vi "Send_Waypoints.vi"() -> ()   [LabVIEW 2009]
uses:
  <vilib>/Instr/_visa.llb/VISA Configure Serial Port (Instr).vi
panel:
  out "Waypoints Received":bool
  out "WRITE BUFFER":string
  out "READ BUFFER":string
  out "error out":errorcluster
  in  "baud rate":u32=115200
  in  "VISA resource name":refnum<visa-resource-name>
  in  "stop":bool
  in  "Request Type":enum16{"Append to End", "Replace List"}(ring)
  in  "Waypoint List":T1(array[cluster])=[{"Latitude"=29.316231, "Longitude"=-81.345678, "Altitude"=100}] {"Longitude" format="%#_15g"; "Latitude" format="%#_15g"}
  in  "Send Waypoints":bool
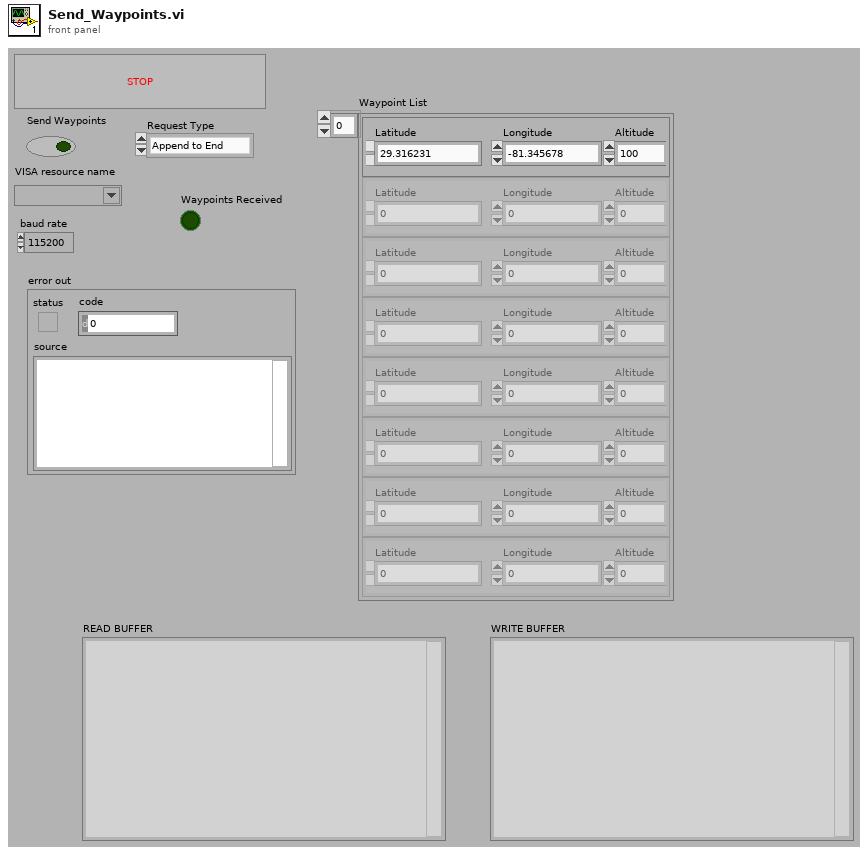
[diagram p1: front panel]
types:
  T1 = cluster{"Latitude":dbl, "Longitude":dbl, "Altitude":u16}[]
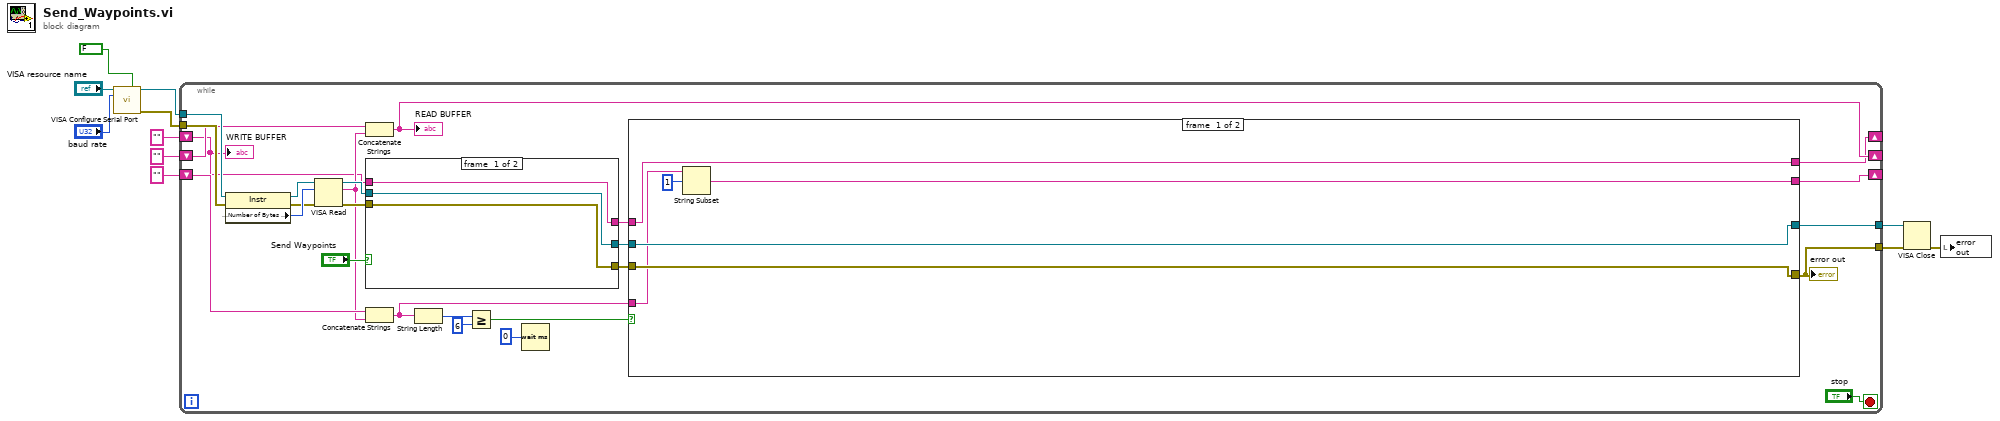
[diagram p0: block diagram]
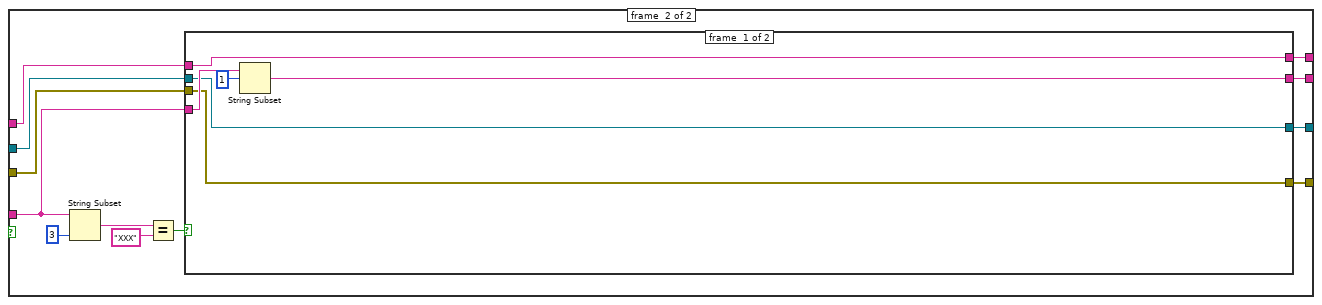
[diagram p2: hidden frame]
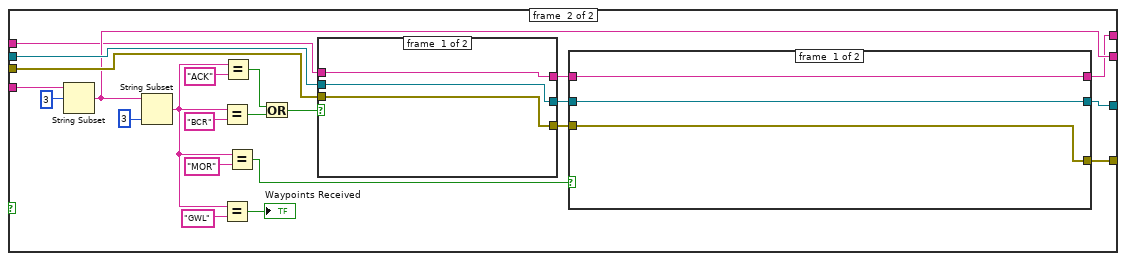
[diagram p3: hidden frame]
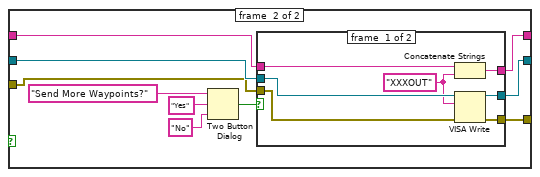
[diagram p4: hidden frame]
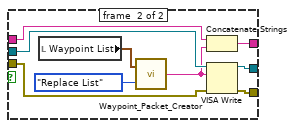
[diagram p5: hidden frame]
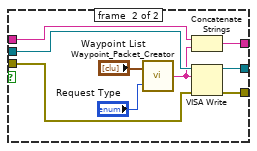
[diagram p6: hidden frame]
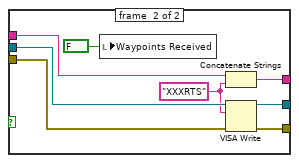
[diagram p7: hidden frame]
diagram:
  n1 = call-poly "VISA Configure Serial Port"("VISA resource name"="VISA resource name", "Enable Termination\nChar (T)"=FALSE ("Enable Termination\nChar (T)"), "baud rate (9600)"="baud rate") -> ("VISA resource name out"=w11:refnum<visa-resource-name>, "error out"=w7:errorcluster)  [unwired: 11 in]
  n2 = while {
    tunnel: w11 -> [w35]
    tunnel: w7 -> [w34]
    shift-right: [w24] -> _
    shift-left: "" -> [w30]
    tunnel: [w21] -> w5
    tunnel: [w20] -> w4
    shift-right: [w15] -> _
    shift-left: "" -> [w17]
    shift-right: [w12] -> _
    shift-left: "" -> [w14]
    stop <- "stop" stop-if-true
    n3 = property class="Instr"(reference=w35, error in=w34) -> (reference out=w33:refnum<visa-resource-name>, error out=w31:errorcluster, "Serial Settings:Number of Bytes at Serial Port"=w32:u32)
    n4 = VISA Read(VISA resource name=w33, byte count=w32, error in (no error)=w31) -> (VISA resource name out=w29:refnum<visa-resource-name>, read buffer=w16:string, error out=w28:errorcluster)  [unwired: 1 out]
    n5 = Concatenate Strings(w17, w16) -> (w15:string)
    "READ BUFFER" <- w15
    n6 = case shown="True" "Send Waypoints" {
      tunnel: w29 -> [w128 w136]
      tunnel: w28 -> [w127 w135]
      tunnel: [w127 w134] -> w22
      tunnel: [w128 w133] -> w23
      tunnel: w14 -> [w126 w131]
      tunnel: [w126 w130] -> w13
      frame #0 {
      }
      frame #1 {
        w132 = "XXXRTS" ("write buffer")
        n7 = local write "Waypoints Received"(FALSE ("Waypoints Received")) -> ()
        n8 = Concatenate Strings(w131, w132) -> (w130:string)
        n9 = VISA Write(VISA resource name=w136, write buffer=w132, error in (no error)=w135) -> (VISA resource name out=w133:refnum<visa-resource-name>, error out=w134:errorcluster)  [unwired: 1 out]
      }
    }
    n10 = Concatenate Strings(w30, w16) -> (w18:string)
    n11 = String Length(string=w18) -> (length=w27:i32)
    n12 = Greater Or Equal?(x=w27, y=6) -> (x >= y?=w25:bool)
    n13 = Wait (ms)(milliseconds to wait=u32 0) -> ()  [unwired: 1 out]
    n14 = case shown="True" w25 {
      tunnel: w18 -> [w41 w51]
      tunnel: [w40 w50] -> w24
      tunnel: w23 -> [w43 w49]
      tunnel: w22 -> [w42 w48]
      tunnel: [w43 w47] -> w21
      tunnel: [w42 w46] -> w20
      tunnel: w13 -> [w38 w45]
      tunnel: [w38 w44] -> w12
      frame #0 {
        n15 = String Subset(string=w41, offset (0)=1 ("length (rest)")) -> (substring=w40:string)  [unwired: 1 in]
      }
      frame #1 {
        n16 = String Subset(string=w51, length (rest)=3 ("length (rest)")) -> (substring=w54:string)  [unwired: 1 in]
        n17 = Equal?(x=w54, y="XXX") -> (x = y?=w52:bool)
        n18 = case shown="True" w52 {
          tunnel: w51 -> [w61 w80]
          tunnel: [w59 w69] -> w50
          tunnel: w49 -> [w58 w78]
          tunnel: w48 -> [w57 w77]
          tunnel: [w58 w71] -> w47
          tunnel: [w57 w70] -> w46
          tunnel: w45 -> [w56 w68]
          tunnel: [w56 w66] -> w44
          frame #0 {
            n19 = String Subset(string=w61, offset (0)=1) -> (substring=w59:string)  [unwired: 1 in]
          }
          frame #1 {
            n20 = String Subset(string=w80, offset (0)=3) -> (substring=w69:string)  [unwired: 1 in]
            n21 = String Subset(string=w69, length (rest)=3 ("length (rest)")) -> (substring=w64:string)  [unwired: 1 in]
            n22 = Equal?(x=w64, y="BCR") -> (x = y?=w63:bool)
            n23 = Equal?(x=w64, y="GWL") -> (x = y?=→"Waypoints Received":bool)
            n24 = Equal?(x=w64, y="ACK") -> (x = y?=w76:bool)
            n25 = Equal?(x=w64, y="MOR") -> (x = y?=w74:bool)
            n26 = Or(x=w76, y=w63) -> (x .or. y?=w75:bool)
            n27 = case shown="True" w75 {
              tunnel: w78 -> [w116 w123]
              tunnel: w77 -> [w115 w122]
              tunnel: [w116 w121] -> w73
              tunnel: [w115 w120] -> w72
              tunnel: w68 -> [w114 w119]
              tunnel: [w114 w117] -> w67
              frame #0 {
              }
              frame #1 {
                n28 = call "Waypoint_Packet_Creator.vi"("Request Type"="Request Type", "Waypoint List"="Waypoint List") -> ("Waypoint Packet"=w118:string)
                n29 = Concatenate Strings(w119, w118) -> (w117:string)
                n30 = VISA Write(VISA resource name=w123, write buffer=w118, error in (no error)=w122) -> (VISA resource name out=w121:refnum<visa-resource-name>, error out=w120:errorcluster)  [unwired: 1 out]
              }
            }
            n31 = case shown="True" w74 {
              tunnel: w73 -> [w86 w93]
              tunnel: w72 -> [w87 w92]
              tunnel: [w86 w91] -> w71
              tunnel: [w87 w90] -> w70
              tunnel: w67 -> [w85 w89]
              tunnel: [w85 w88] -> w66
              frame #0 {
              }
              frame #1 {
                n32 = Two Button Dialog(message="Send More Waypoints?", 1:"No" ("F button name (\"Cancel\")"), 2:"Yes" ("T button name (\"OK\")")) -> (T button?=w94:bool)
                n33 = case shown="False" w94 {
                  tunnel: w93 -> [w104 w113]
                  tunnel: w92 -> [w103 w112]
                  tunnel: [w102 w111] -> w91
                  tunnel: [w101 w110] -> w90
                  tunnel: w89 -> [w99 w106]
                  tunnel: [w98 w105] -> w88
                  frame #0 {
                    w100 = "XXXOUT" ("write buffer")
                    n34 = Concatenate Strings(w99, w100) -> (w98:string)
                    n35 = VISA Write(VISA resource name=w104, write buffer=w100, error in (no error)=w103) -> (VISA resource name out=w102:refnum<visa-resource-name>, error out=w101:errorcluster)  [unwired: 1 out]
                  }
                  frame #1 {
                    n36 = local read "Waypoint List"() -> (w109:T1)
                    n37 = call "Waypoint_Packet_Creator.vi"("Request Type"=enum16{"Append to End", "Replace List"}."Replace List", "Waypoint List"=w109) -> ("Waypoint Packet"=w107:string)
                    n38 = Concatenate Strings(w106, w107) -> (w105:string)
                    n39 = VISA Write(VISA resource name=w113, write buffer=w107, error in (no error)=w112) -> (VISA resource name out=w111:refnum<visa-resource-name>, error out=w110:errorcluster)  [unwired: 1 out]
                  }
                }
              }
            }
          }
        }
      }
    }
    "error out" <- w20
    "WRITE BUFFER" <- w14
  }
  n40 = VISA Close(VISA resource name=w5, error in (no error)=w4) -> (error out=w3:errorcluster)
  n41 = local write "error out"(w3) -> ()
